vi "Spindle Speed.vi"(8 "error in (no error)":errorcluster, 11 "Cluster":T1) -> (0 "error out":errorcluster, 3 "number":i32)   [LabVIEW 2021]
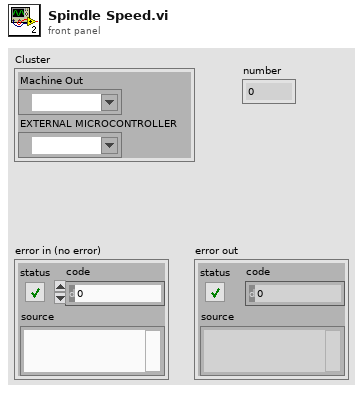
[diagram p1: front panel]
types:
  T1 = cluster{"Machine Out":refnum<visa-resource-name>, "EXTERNAL MICROCONTROLLER":refnum<visa-resource-name>}
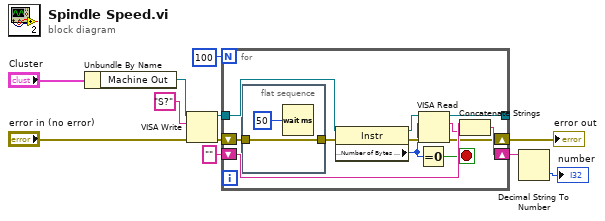
[diagram p0: block diagram]
diagram:
  n1 = Unbundle By Name("Cluster") -> ("Machine Out"=w9:refnum<visa-resource-name>)
  n2 = VISA Write(VISA resource name=w9, write buffer="S?", error in (no error)="error in (no error)") -> (VISA resource name out=w6:refnum<visa-resource-name>, error out=w5:errorcluster)  [unwired: 1 out]
  n3 = for {
    N: 100 -> [_]
    tunnel: w6 -> [w20]
    shift-right: [w23] -> w2
    shift-left: "" -> [w22]
    shift-right: [w17] -> w11
    shift-left: w5 -> [w15]
    tunnel: [w12] -> _
    stop <- w13 stop-if-true
    n4 = flat-sequence {
      tunnel: w15 -> [w24]
      tunnel: [w24] -> w14
      frame #0 {
        n5 = Wait (ms)(milliseconds to wait=u32 50) -> ()  [unwired: 1 out]
      }
    }
    n6 = property class="Instr"(reference=w20, error in=w14) -> (reference out=w16:refnum<visa-resource-name>, error out=w21:errorcluster, "Serial Settings:Number of Bytes at Serial Port"=w18:u32)
    n7 = Equal To 0?(x=w18) -> (x = 0?=w13:bool)
    n8 = VISA Read(VISA resource name=w16, byte count=w18, error in (no error)=w21) -> (VISA resource name out=w12:refnum<visa-resource-name>, read buffer=w19:string, error out=w17:errorcluster)  [unwired: 1 out]
    n9 = Concatenate Strings(w22, w19) -> (w23:string)
  }
  "error out" <- w11
  n10 = Decimal String To Number(string=w2) -> (number=→"number":i32)  [unwired: 2 in, 1 out]
